vi "SubVI_Filter_Impedances.vi"(8 "error in (no error)":errorcluster, 9 "Resampling rate":dbl, 10 "Interpolant Size":dbl, 11 "Constant Impedances In":T1) -> (0 "error out":errorcluster, 3 "Filtered Impedances Out":T2)   [LabVIEW 2020]
uses:
  <extravilib>/ChannelInstances/Lossy Stream-a[.,.](dbl)/)Channel.ctl
  <extravilib>/ChannelInstances/Stream-a[.](dbl)/)Channel.ctl
  <vilib>/Analysis/3filter.llb/Filter Passband Type.ctl
  <extravilib>/ChannelInstances/Stream-a[.](dbl)/EndpointRead.vi
  <extravilib>/ChannelInstances/Lossy Stream-a[.,.](dbl)/Endpoint.vi
  Global 1.vi
  <extravilib>/ChannelInstances/Stream-a[.](dbl)/)Channel.vi
  <resource>/ChannelSupport/_ChannelSupport/WaitIfNeeded.vi
  <extravilib>/ChannelInstances/Lossy Stream-a[.,.](dbl)/)Channel.vi
  <extravilib>/ChannelInstances/Lossy Stream-a[.,.](dbl).lvlib
  <extravilib>/ChannelInstances/Stream-a[.](dbl).lvlib
  <vilib>/Analysis/NI_AALBase.lvlib
  <vilib>/ptbypt/NI_PtbyPt.lvlib
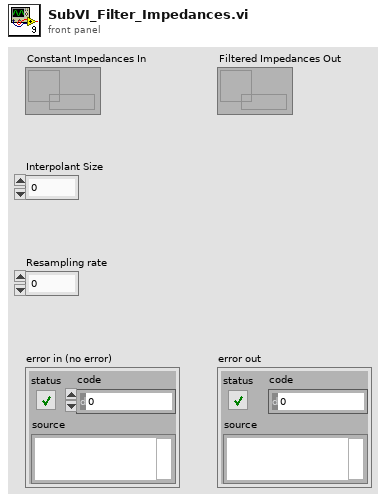
[diagram p1: front panel]
types:
  T1 = typedef "Stream-a[.](dbl).lvlib/)Channel.ctl" = refnum<queue>
  T2 = typedef "Lossy Stream-a[.,.](dbl).lvlib/)Channel.ctl" = refnum<queue>
  T3 = typedef "NI_AALBase.lvlib/Filter Passband Type.ctl" = enum32{"Lowpass", "Highpass", "Bandpass", "Bandstop"}
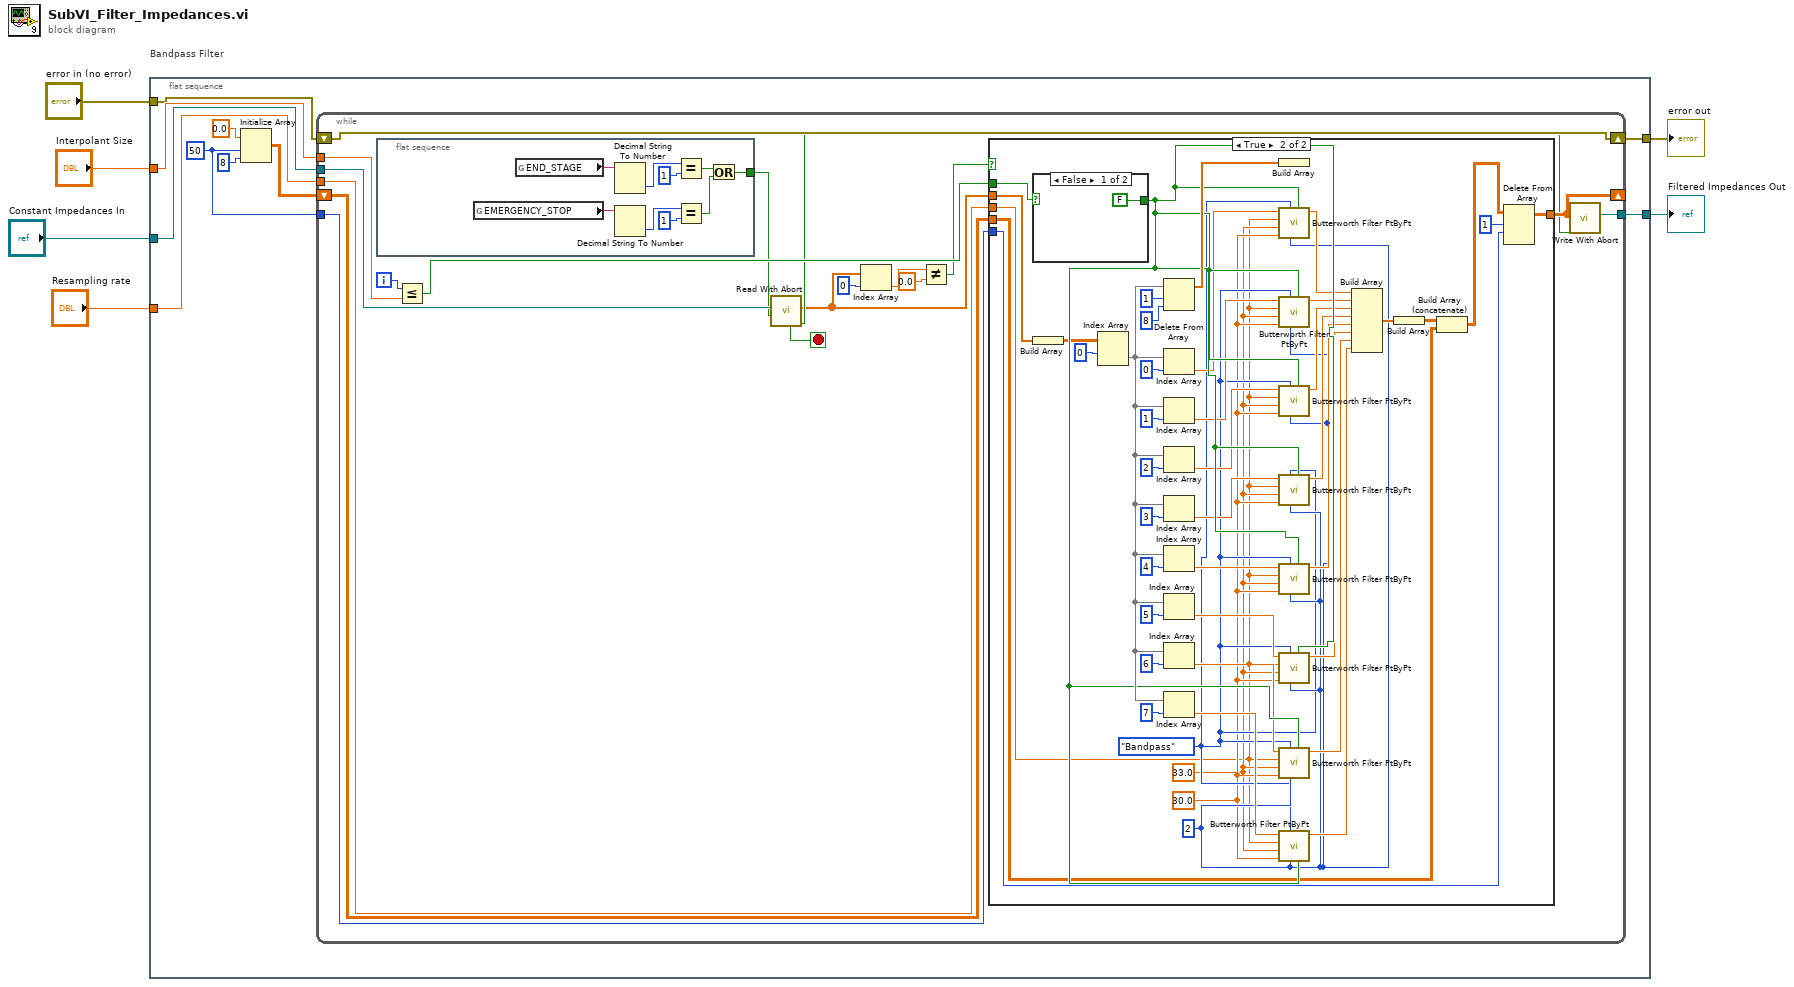
[diagram p0: block diagram]
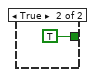
[diagram p3: hidden frame]
diagram:
  n1 = flat-sequence "Bandpass Filter" {
    tunnel: "Constant Impedances In" -> [w16]
    tunnel: "Interpolant Size" -> [w15]
    tunnel: [w14] -> w3
    tunnel: [w10] -> w4
    tunnel: "error in (no error)" -> [w8]
    tunnel: "Resampling rate" -> [w7]
    frame #0 {
      w9 = 50 ("dimension size")
      n2 = Initialize Array(0.0 ("element"), w9, 8 ("dimension size")) -> (w12:dbl[][])
      n3 = while {
        tunnel: w7 -> [w33]
        tunnel: w16 -> [w32]
        tunnel: w15 -> [w30]
        shift-right: [w28] -> w14
        shift-left: w8 -> [w28]
        shift-right: [w25] -> _
        shift-left: w12 -> [w27]
        tunnel: w9 -> [w26]
        tunnel: [w23] -> w10
        i -> [w31]
        stop <- w24 stop-if-true
        n4 = flat-sequence {
          tunnel: [w34] -> w17
          frame #0 {
            n5 = global read "Global 1.vi" "EMERGENCY_STOP"() -> (w37:string)
            n6 = global read "Global 1.vi" "END_STAGE"() -> (w42:string)
            n7 = Decimal String To Number(string=w42) -> (number=w41:i32)  [unwired: 2 in, 1 out]
            n8 = Decimal String To Number(string=w37) -> (number=w39:i32)  [unwired: 2 in, 1 out]
            n9 = Equal?(x=w41, y=1) -> (x = y?=w35:bool)
            n10 = Equal?(x=w39, y=1) -> (x = y?=w36:bool)
            n11 = Or(x=w35, y=w36) -> (x .or. y?=w34:bool)
          }
        }
        n12 = Less Or Equal?(x=w31, y=w30) -> (x <= y?=w29:bool)
        n13 = call <extravilib>:"Read With Abort.vi"("abort"=w17, "channel"=w32) -> ("element"=w22:dbl[], "aborted?"=w24:bool)  [unwired: 4 in, 4 out]
        n14 = Index Array(array=w22, index=0) -> (element=w20:dbl)
        n15 = Not Equal?(x=w20, y=0.0) -> (x != y?=w18:bool)
        n16 = case shown="True" w18 {
          tunnel: w33 -> [_ w54]
          tunnel: w22 -> [_ w52]
          tunnel: w29 -> [_ w50]
          tunnel: w27 -> [w43 w49]
          tunnel: w26 -> [_ w47]
          tunnel: [w43 w45] -> w25
          frame False {
          }
          frame True {
            w65 = 2 ("order")
            w63 = 30.0 ("low cutoff freq: fl")
            w62 = 33.0 ("high cutoff freq: fh")
            w64 = Filter_Passband_Type."Bandpass" ("filter type")
            n17 = case shown="False" w50 {
              tunnel: [FALSE TRUE] -> w85
              frame False {
              }
              frame True {
              }
            }
            n18 = Build Array(w52) -> (w51:dbl[][])
            n19 = Index Array(array=w51, index (row)=0) -> (element=w87:dbl[])  [unwired: 1 in]
            n20 = Delete From Array(array=w87, length=1, index=8) -> (array with subset deleted=w88:dbl[])  [unwired: 1 out]
            n21 = Index Array(array=w87, index=0) -> (element=w69:dbl)
            n22 = Index Array(array=w87, index=1) -> (element=w70:dbl)
            n23 = Index Array(array=w87, index=2) -> (element=w71:dbl)
            n24 = Index Array(array=w87, index=3) -> (element=w72:dbl)
            n25 = Index Array(array=w87, index=4) -> (element=w73:dbl)
            n26 = Index Array(array=w87, index=5) -> (element=w74:dbl)
            n27 = Index Array(array=w87, index=6) -> (element=w75:dbl)
            n28 = Index Array(array=w87, index=7) -> (element=w76:dbl)
            n29 = Build Array(w88) -> ()  [unwired: 1 out]
            n30 = call <vilib>:"Butterworth Filter PtByPt.vi"("initialize"=w85, "order"=w65, "filter type"=w64, "low cutoff freq: fl"=w63, "high cutoff freq: fh"=w62, "sampling freq: fs"=w54, "x"=w69) -> ("Filtered x"=w77:dbl)  [unwired: 2 in, 1 out]
            n31 = call <vilib>:"Butterworth Filter PtByPt.vi"("initialize"=w85, "order"=w65, "filter type"=w64, "low cutoff freq: fl"=w63, "high cutoff freq: fh"=w62, "sampling freq: fs"=w54, "x"=w70) -> ("Filtered x"=w78:dbl)  [unwired: 2 in, 1 out]
            n32 = call <vilib>:"Butterworth Filter PtByPt.vi"("initialize"=w85, "order"=w65, "filter type"=w64, "low cutoff freq: fl"=w63, "high cutoff freq: fh"=w62, "sampling freq: fs"=w54, "x"=w71) -> ("Filtered x"=w79:dbl)  [unwired: 2 in, 1 out]
            n33 = call <vilib>:"Butterworth Filter PtByPt.vi"("initialize"=w85, "order"=w65, "filter type"=w64, "low cutoff freq: fl"=w63, "high cutoff freq: fh"=w62, "sampling freq: fs"=w54, "x"=w72) -> ("Filtered x"=w80:dbl)  [unwired: 2 in, 1 out]
            n34 = call <vilib>:"Butterworth Filter PtByPt.vi"("initialize"=w85, "order"=w65, "filter type"=w64, "low cutoff freq: fl"=w63, "high cutoff freq: fh"=w62, "sampling freq: fs"=w54, "x"=w73) -> ("Filtered x"=w81:dbl)  [unwired: 2 in, 1 out]
            n35 = call <vilib>:"Butterworth Filter PtByPt.vi"("initialize"=w85, "order"=w65, "filter type"=w64, "low cutoff freq: fl"=w63, "high cutoff freq: fh"=w62, "sampling freq: fs"=w54, "x"=w74) -> ("Filtered x"=w82:dbl)  [unwired: 2 in, 1 out]
            n36 = call <vilib>:"Butterworth Filter PtByPt.vi"("initialize"=w85, "order"=w65, "filter type"=w64, "low cutoff freq: fl"=w63, "high cutoff freq: fh"=w62, "sampling freq: fs"=w54, "x"=w75) -> ("Filtered x"=w83:dbl)  [unwired: 2 in, 1 out]
            n37 = call <vilib>:"Butterworth Filter PtByPt.vi"("initialize"=w85, "order"=w65, "filter type"=w64, "low cutoff freq: fl"=w63, "high cutoff freq: fh"=w62, "sampling freq: fs"=w54, "x"=w76) -> ("Filtered x"=w84:dbl)  [unwired: 2 in, 1 out]
            n38 = Build Array(w77, w78, w79, w80, w81, w82, w83, w84) -> (w86:dbl[])
            n39 = Build Array(w86) -> (w44:dbl[][])
            n40 = Build Array (concatenate)(w44, w49) -> (w48:dbl[][])
            n41 = Delete From Array(array=w48, length=1, index (row)=w47) -> (array with subset deleted=w45:dbl[][])  [unwired: 1 in, 1 out]
          }
        }
        n42 = call <extravilib>:"Write With Abort.vi"("abort"=w24, "element"=w25) -> ("channel"=w23:T2)  [unwired: 6 in, 3 out]
      }
    }
  }
  "Filtered Impedances Out" <- w4
  "error out" <- w3
